vi "Add Range.vi"(8 "error in (no error)":errorcluster caption="错误输入（无错误）", 9 "Values":string[](array[string]), 10 "Keys":string[](array[string]), 11 "Dictionary In":refnum<class "Dictionary.lvclass"> caption="DNL_LabVIEW Object in") -> (0 "error out":errorcluster caption="错误输出", 1 "Key Exist?":bool, 3 "Dictionary Out":refnum<class "Dictionary.lvclass"> caption="DNL_LabVIEW Object out")   [LabVIEW 2012, in "Dictionary.lvclass"]
uses:
  Dictionary.lvclass
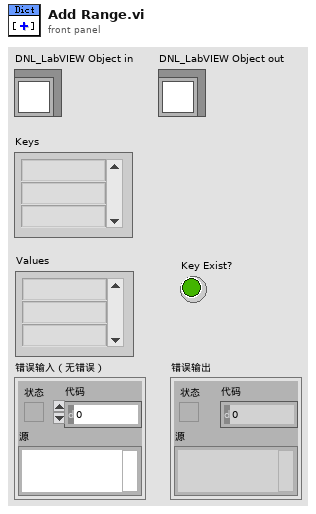
[diagram p1: front panel]
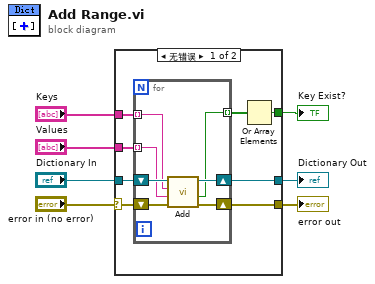
[diagram p0: block diagram]
diagram:
  n1 = case shown="无错误" "error in (no error)" {
    selector: "error in (no error)" -> [w11 w24]
    tunnel: [w10 w24] -> w6
    tunnel: [w12 w23] -> w4
    tunnel: "Dictionary In" -> [w15 w23]
    tunnel: "Values" -> [w13 _]
    tunnel: "Keys" -> [w14 _]
    tunnel: [w8 _] -> w1
    frame No Error {
      n2 = for {
        shift-right: [w19] -> w12
        shift-left: w15 -> [w22]
        tunnel: w14 -> [w21] mode=indexing
        tunnel: w13 -> [w20] mode=indexing
        tunnel: [w18] -> w9 mode=indexing
        shift-right: [w16] -> w10
        shift-left: w11 -> [w17]
        n3 = call "Add.vi"("error in (no error)"=w17, "Value"=w20, "Key"=w21, "Dictionary In"=w22) -> ("error out"=w16:errorcluster, "Key Exist?"=w18:bool, "Dictionary Out"=w19:refnum<class "Dictionary.lvclass">)  [unwired: 5 in]
      }
      n4 = Or Array Elements(Boolean array=w9) -> (logical OR=w8:bool)
    }
    frame Error {
    }
  }
  "error out" <- w6
  "Dictionary Out" <- w4
  "Key Exist?" <- w1
